vi "MT Measure Burst Timing.vi"(0 "input complex waveform":T2={"t0"=0.0, "dt"=1.0, "Y"=[]} {"Y" format="%.3f"; "dt" format="%^.2e"; "t0" format="%.4f"}, 1 "impairment measurement window":T1={"start index (samples)"=0, "width (samples)"=100}, 5 "upper mask (dB)":dbl[](array[numeric]) format="%.2f", 7 "ideal power curve (dB)":dbl[](array[numeric]) format="%.2f", 9 "lower mask (dB)":dbl[](array[numeric]) format="%.2f", 11 "error in (no error)":errorcluster) -> (3 "amplitude droop (dB)":dbl format="%.2f", 4 "pass?":bool, 6 "first error sample index":i32, 8 "correlated burst index (samples)":i32, 10 "crest factor (dB)":dbl format="%.2f", 15 "error out":errorcluster)   [LabVIEW 2020, in "niDMT.lvlib"]
doc: "Locates a burst within the <B>input complex waveform</B> with peaks correlating to the input <B>ideal power curve</B>."
uses:
  <vilib>/addons/Modulation/niDMT.lvlib
  <vilib>/addons/Modulation/Analog/controls/Complex Data Waveform.ctl
  <vilib>/Analysis/baseanly.llb/Mean (DBL).vi
  <vilib>/Analysis/2dsp.llb/1D Cross Correlation (DBL).vi
  <vilib>/addons/Modulation/niAMT.lvlib
  <vilib>/Analysis/NI_AALPro.lvlib
  <vilib>/Analysis/NI_AALBase.lvlib
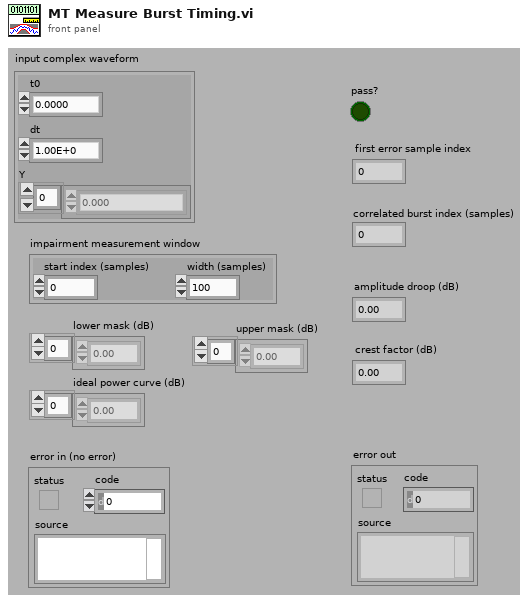
[diagram p1: front panel]
types:
  T1 = cluster{"start index (samples)":i32, "width (samples)":i32}
  T2 = typedef "niAMT.lvlib/Complex Data Waveform.ctl" = cluster{"t0":dbl, "dt":dbl, "Y":cdb[]}
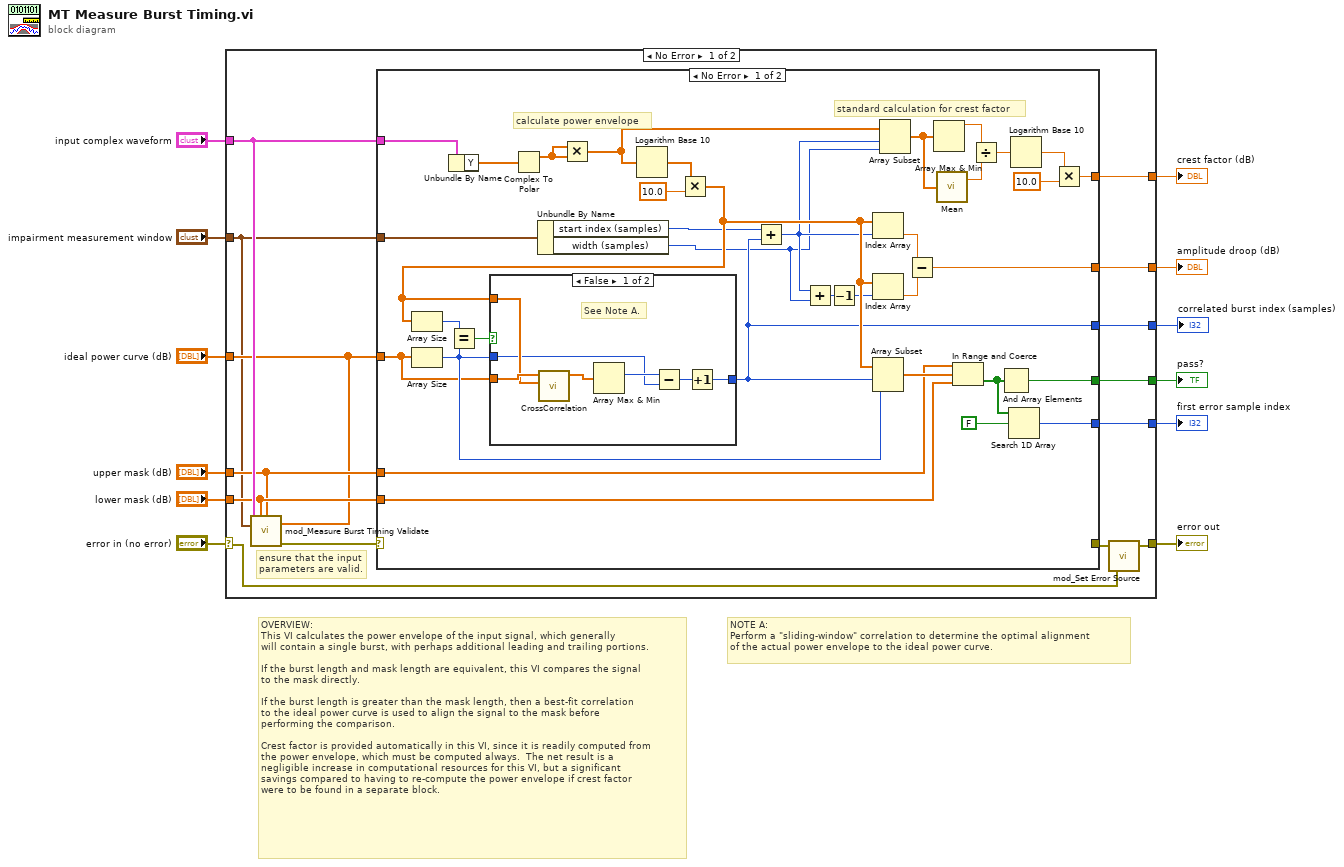
[diagram p0: block diagram]
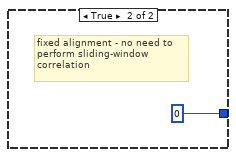
[diagram p2: hidden frame]
diagram:
  # "OVERVIEW:\nThis VI calculates the power envelope of the input signal, which generally\nwill contain a single burst, with perhaps additional leading and trailing portions.\n\nIf the burst length and mask length are equivalent, this VI compares the signal\nto the mask directly.\n\nIf the burst length is greater than the mask length, then a best-fit correlation\nto the ideal power curve is used to align the signal to the mask before\nperforming the comparison.\n\nCrest factor is provided automatically in this VI, since it is readily computed from\nthe power envelope, which must be computed always.  The net result is a \nnegligible increase in computational resources for this VI, but a significant\nsavings compared to having to re-compute the power envelope if crest factor\nwere to be found in a separate block."
  # "NOTE A:\nPerform a \"sliding-window\" correlation to determine the optimal alignment\nof the actual power envelope to the ideal power curve."
  n1 = case shown="No Error" "error in (no error)" {
    selector: "error in (no error)" -> [w13 w71]
    tunnel: "input complex waveform" -> [w20 _]
    tunnel: "ideal power curve (dB)" -> [w17 _]
    tunnel: [w25 _] -> w9
    tunnel: "impairment measurement window" -> [w16 _]
    tunnel: [w24 _] -> w7
    tunnel: "upper mask (dB)" -> [w18 _]
    tunnel: "lower mask (dB)" -> [w19 _]
    tunnel: [w23 _] -> w4
    tunnel: [w22 _] -> w3
    tunnel: [w21 _] -> w2
    tunnel: [w14 w71] -> w1
    frame No Error {
      # "ensure that the input parameters are valid."
      n2 = call <vilib>:"mod_Measure Burst Timing Validate.vi"("input complex waveform"=w20, "Lower Mask, dB"=w19, "upper mask (dB)"=w18, "ideal power curve (dB)"=w17, "Impairment Measurement Window"=w16) -> ("error out"=w26:errorcluster)  [unwired: 10 out]
      n3 = case shown="No Error" w26 {
        selector: w26 -> [_ w70]
        tunnel: w20 -> [w61 _]
        tunnel: w17 -> [w38 _]
        tunnel: [w49 _] -> w25
        tunnel: w16 -> [w48 _]
        tunnel: [w45 _] -> w24
        tunnel: w18 -> [w36 _]
        tunnel: w19 -> [w37 _]
        tunnel: [w42 _] -> w23
        tunnel: [w31 _] -> w22
        tunnel: [w35 _] -> w21
        tunnel: [_ w70] -> w15
        frame No Error {
          # "standard calculation for crest factor"
          # "calculate power envelope"
          n4 = Array Size(array=w38) -> (size(s)=w44:i32)
          n5 = Unbundle By Name(w61) -> ("Y"=w56:cdb[])
          n6 = Complex To Polar(r * e^(i*theta)=w56) -> (r=w60:dbl[])  [unwired: 1 out]
          n7 = Unbundle By Name(w48) -> ("start index (samples)"=w32:i32, "width (samples)"=w29:i32)
          n8 = Multiply(x=w60, y=w60) -> (x*y=w33:dbl[])
          n9 = Logarithm Base 10(1:w33) -> (0:w59:dbl[])
          n10 = Multiply(x=w59, y=10.0) -> (x*y=w39:dbl[])
          n11 = Array Size(array=w39) -> (size(s)=w55:i32)
          n12 = Equal?(x=w55, y=w44) -> (x = y?=w57:bool)
          n13 = case shown="False" w57 {
            tunnel: w39 -> [w67 _]
            tunnel: w38 -> [w68 _]
            tunnel: [w64 0] -> w35
            tunnel: w44 -> [w63 _]
            frame False {
              # "See Note A."
              n14 = call-poly <vilib>:"CrossCorrelation.vi"("Y"=w67, "X"=w68) -> ("Rxy"=w62:dbl[])  [unwired: 2 in, 7 out]
              n15 = Array Max & Min(array=w62) -> (max index (indices)=w66:i32)  [unwired: 3 out]
              n16 = Subtract(x=w66, y=w63) -> (x-y=w65:i32)
              n17 = Increment(x=w65) -> (x+1=w64:i32)
            }
            frame True {
              # "fixed alignment - no need to\nperform sliding-window\ncorrelation"
            }
          }
          n18 = Add(x=w32, y=w35) -> (x+y=w30:i32)
          n19 = Add(x=w30, y=w29) -> (x+y=w28:i32)
          n20 = Decrement(x=w28) -> (x-1=w27:i32)
          n21 = Index Array(array=w39, index=w30) -> (element=w47:dbl)
          n22 = Index Array(array=w39, index=w27) -> (element=w46:dbl)
          n23 = Array Subset(array=w39, index=w35, length=w44) -> (w43:dbl[])
          n24 = Array Subset(array=w33, index=w30, length=w29) -> (w34:dbl[])
          n25 = Subtract(x=w47, y=w46) -> (x-y=w45:dbl)
          n26 = Array Max & Min(array=w34) -> (max value=w54:dbl)  [unwired: 3 out]
          n27 = call-poly <vilib>:"Mean.vi"("X"=w34) -> ("mean"=w53:dbl)  [unwired: 1 out]
          n28 = In Range and Coerce(upper limit=w36, x=w43, lower limit=w37) -> (In Range?=w41:bool[])  [unwired: 1 out]
          n29 = Divide(x=w54, y=w53) -> (x/y=w50:dbl)
          n30 = And Array Elements(Boolean array=w41) -> (logical AND=w42:bool)
          n31 = Search 1D Array(1D array=w41, element=FALSE) -> (index of element=w31:i32)  [unwired: 1 out]
          n32 = Logarithm Base 10(1:w50) -> (0:w51:dbl)
          n33 = Multiply(x=w51, y=10.0) -> (x*y=w49:dbl)
        }
        frame Error {
        }
      }
      n34 = call <vilib>:"mod_Set Error Source.vi"("initial error in (no error)"=w13, "final error in (no error)"=w15) -> ("error out"=w14:errorcluster)  [unwired: 3 out]
    }
    frame Error {
    }
  }
  "error out" <- w1
  "amplitude droop (dB)" <- w7
  "crest factor (dB)" <- w9
  "first error sample index" <- w3
  "correlated burst index (samples)" <- w2
  "pass?" <- w4
